vi "Match_Pressure STD.vi"(8 "abs?(F)":bool, 9 "분류코드":string, 10 "Cal STD 입력":string[][](array[string]), 11 "Condition in":string[][](array[string])) -> (0 "Cal STD(-)":string[](array[string]), 1 "Dead Weight":string[][](array[string]), 2 "Cal STD(+)":string[](array[string]), 3 "Condition out":string[][](array[string]), 4 "Cal STD(DMM)":string[][](array[string]), 5 "단위":string, 6 "Power Supply?":string, 7 "STD Name":string)   [LabVIEW 2020]
uses:
  Public/Polymorph/Data Class_2D Str.vi
  Public/Polymorph/Sort_2D Str.vi
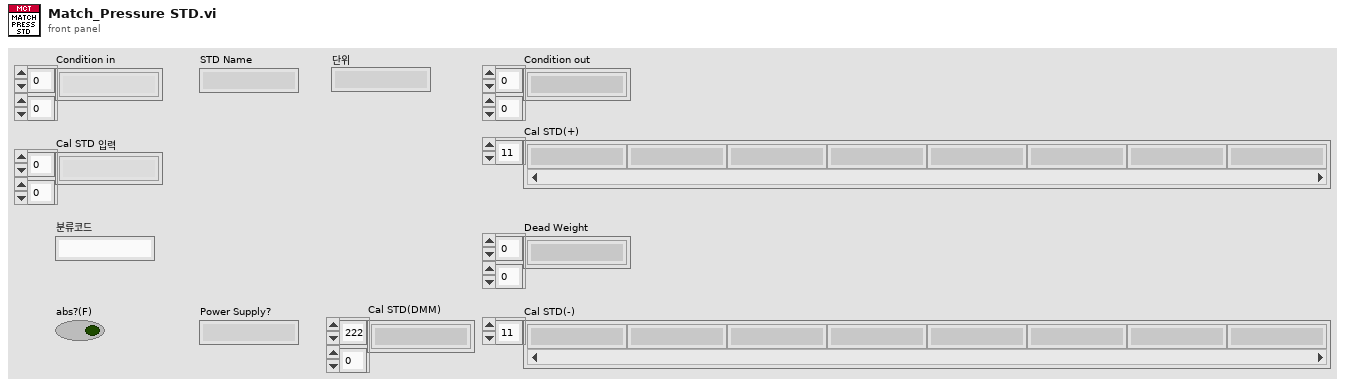
[diagram p1: front panel]
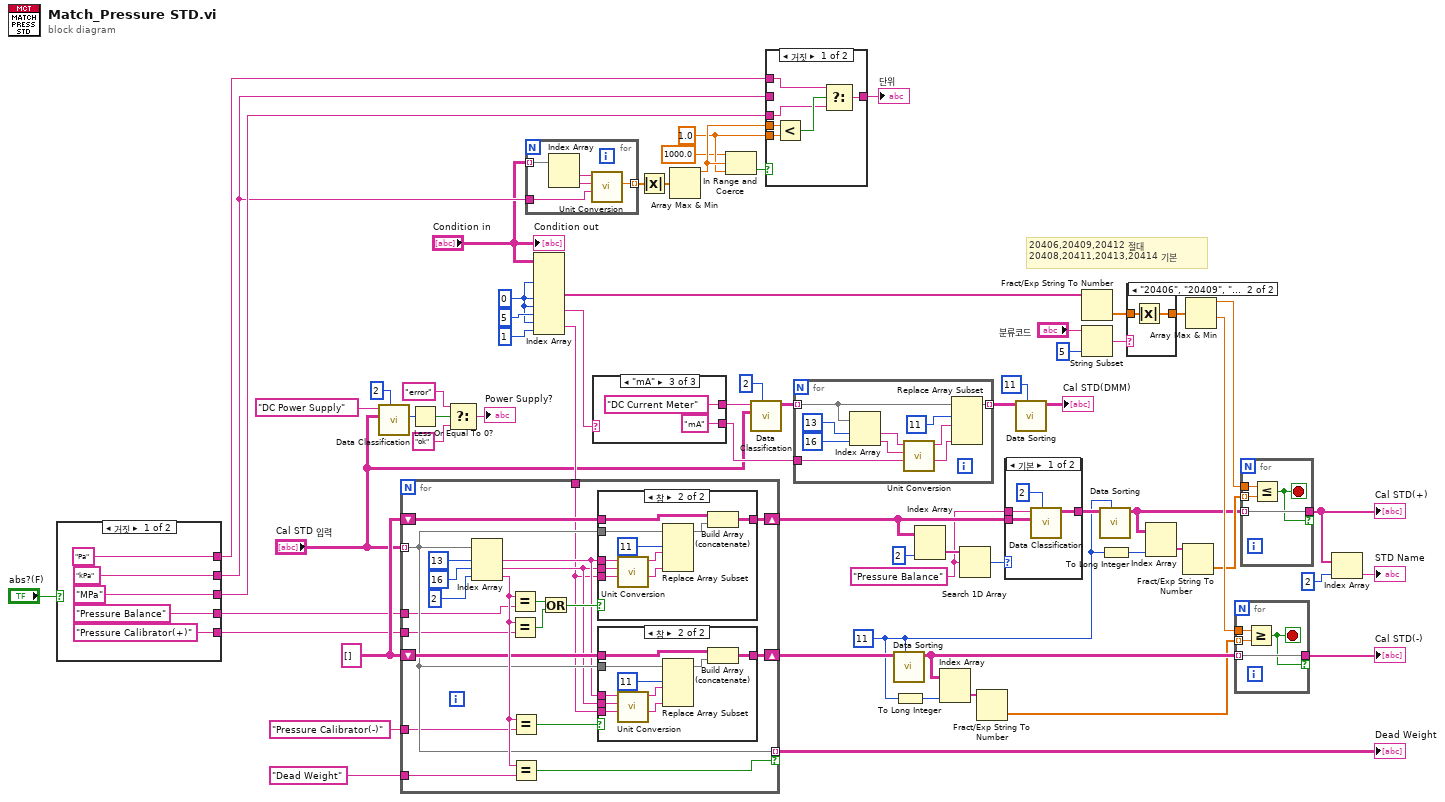
[diagram p0: block diagram]
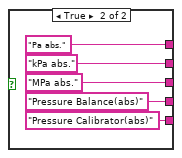
[diagram p2: hidden frame]
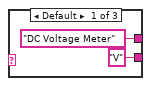
[diagram p4: hidden frame]
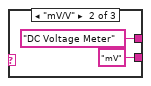
[diagram p5: hidden frame]
diagram:
  w40 = 1.0 ("하위 리미트")
  w2 = "Pressure Balance"
  w8 = u16 11 ("기준열")
  w5 = 0 ("인덱스 (행)")
  w66 = string[][] []
  # "20406,20409,20412 절대\n20408,20411,20413,20414 기본"
  n1 = case shown="거짓" "abs?(F)" {
    tunnel: ["Pressure Balance" "Pressure Balance(abs)"] -> w16
    tunnel: ["Pressure Calibrator(+)" "Pressure Calibrator(abs)"] -> w15
    tunnel: ["kPa" ("환산단위") "kPa abs." ("환산단위")] -> w12
    tunnel: ["Pa" "Pa abs."] -> w14
    tunnel: ["MPa" "MPa abs."] -> w13
    frame False {
    }
    frame True {
    }
  }
  n2 = call-poly "Data Classification.vi"("인덱스"=2, "DATA 입력"="Cal STD 입력", "검색 문자열"="DC Power Supply") -> ("행크기"=w26:i32)  [unwired: 4 in, 4 out]
  n3 = Less Or Equal To 0?(x=w26) -> (x <= 0?=w27:bool)
  n4 = Select(t="error" ("검색 문자열"), s=w27, f="ok") -> (s? t:f=→"Power Supply?":string)
  n5 = for {
    tunnel: "Condition in" -> [w81] mode=indexing
    tunnel: [w78] -> w37 mode=indexing
    tunnel: w12 -> [w77]
    n6 = Index Array(array=w81) -> (element #1=w80:string, element #2=w79:string)  [unwired: 2 in]
    n7 = call "Unit Conversion.vi"("환산단위"=w77, "입력단위"=w79, "입력값"=w80) -> ("환산값 (DBL)"=w78:dbl)  [unwired: 3 in, 5 out]
  }
  n8 = Index Array(array="Condition in", index (col) #1=w5, index (col) #2=w5, index (row) #3=w5, index (col) #3=5 ("비활성화된 인덱스 (열)"), index (row) #4=w5, index (col) #4=1 ("비활성화된 인덱스 (열)")) -> (element #2=w4:string[], element #3=w6:string, element #4=w63:string)  [unwired: 2 in, 1 out]
  n9 = for {
    tunnel: "Cal STD 입력" -> [w89] mode=indexing
    shift-right: [w98] -> w54
    shift-left: w66 -> [w97]
    tunnel: w63 -> [w86]
    tunnel: [w89] -> w65 mode=indexing if=w94
    shift-right: [w91] -> w57
    shift-left: w66 -> [w92]
    tunnel: w16 -> [w85]
    tunnel: w15 -> [w84]
    tunnel: "Pressure Calibrator(-)" -> [w83]
    tunnel: "Dead Weight" -> [w82]
    n10 = Index Array(array=w89, index #1=13 ("인덱스"), index #2=16 ("인덱스"), index #3=2 ("인덱스")) -> (element #1=w88:string, element #2=w87:string, element #3=w93:string)
    n11 = Equal?(x=w93, y=w85) -> (x = y?=w101:bool)
    n12 = Equal?(x=w93, y=w84) -> (x = y?=w100:bool)
    n13 = Equal?(x=w93, y=w83) -> (x = y?=w90:bool)
    n14 = Equal?(x=w93, y=w82) -> (x = y?=w94:bool)
    n15 = Or(x=w101, y=w100) -> (x .or. y?=w99:bool)
    n16 = case shown="참" w99 {
      tunnel: w89 -> [_ w119]
      tunnel: [w114 w124] -> w98
      tunnel: w97 -> [w114 w123]
      tunnel: w88 -> [_ w122]
      tunnel: w87 -> [_ w121]
      tunnel: w86 -> [_ w120]
      frame False {
      }
      frame True {
        n17 = call "Unit Conversion.vi"("환산단위"=w120, "입력단위"=w121, "입력값"=w122) -> ("환산단위"=w117:string, "환산값 (string)"=w118:string)  [unwired: 3 in, 4 out]
        n18 = Replace Array Subset(array=w119, new element #1=w118, index #1=11 ("인덱스"), new element #2=w117) -> (w115:string[])  [unwired: 1 in]
        n19 = Build Array (concatenate)(w123, w115) -> (w124:string[][])
      }
    }
    n20 = case shown="참" w90 {
      tunnel: w89 -> [_ w109]
      tunnel: [w103 w104] -> w91
      tunnel: w92 -> [w103 w113]
      tunnel: w88 -> [_ w112]
      tunnel: w87 -> [_ w111]
      tunnel: w86 -> [_ w110]
      frame False {
      }
      frame True {
        n21 = call "Unit Conversion.vi"("환산단위"=w110, "입력단위"=w111, "입력값"=w112) -> ("환산단위"=w107:string, "환산값 (string)"=w108:string)  [unwired: 3 in, 4 out]
        n22 = Replace Array Subset(array=w109, new element #1=w108, index #1=11 ("인덱스"), new element #2=w107) -> (w105:string[])  [unwired: 1 in]
        n23 = Build Array (concatenate)(w113, w105) -> (w104:string[][])
      }
    }
  }
  "Dead Weight" <- w65
  n24 = case shown="\"mA\"" w6 {
    tunnel: ["DC Voltage Meter" ("검색 문자열") "DC Voltage Meter" ("검색 문자열") "DC Current Meter" ("검색 문자열")] -> w34
    tunnel: ["V" "mV" "mA"] -> w32
    frame Default {
    }
    frame "mV/V" {
    }
    frame "mA" {
    }
  }
  n25 = Absolute Value(x=w37) -> (abs(x)=w42:dbl[])
  n26 = Array Max & Min(array=w42) -> (max value=w41:dbl)  [unwired: 3 out]
  n27 = In Range and Coerce(upper limit=1000.0 ("상위 리미트"), x=w41, lower limit=w40) -> (In Range?=w39:bool)  [unwired: 1 out]
  n28 = call-poly "Data Classification.vi"("인덱스"=2, "DATA 입력"="Cal STD 입력", "검색 문자열"=w34) -> ("DATA 출력"=w33:string[][])  [unwired: 4 in, 4 out]
  n29 = case shown="거짓" w39 {
    tunnel: [w133 w137] -> w36
    tunnel: w40 -> [w136 _]
    tunnel: w41 -> [w135 _]
    tunnel: w14 -> [w132 _]
    tunnel: w13 -> [w131 _]
    tunnel: w12 -> [_ w137]
    frame False {
      n30 = Less?(x=w135, y=w136) -> (x < y?=w134:bool)
      n31 = Select(t=w132, s=w134, f=w131) -> (s? t:f=w133:string)
    }
    frame True {
    }
  }
  "단위" <- w36
  n32 = for {
    tunnel: w33 -> [w143] mode=indexing
    tunnel: [w142] -> w30 mode=indexing
    tunnel: w32 -> [w147]
    n33 = Index Array(array=w143, index #1=13 ("인덱스"), index #2=16 ("인덱스")) -> (element #1=w145:string, element #2=w138:string)
    n34 = call "Unit Conversion.vi"("환산단위"=w147, "입력단위"=w138, "입력값"=w145) -> ("환산단위"=w139:string, "환산값 (string)"=w140:string)  [unwired: 3 in, 4 out]
    n35 = Replace Array Subset(array=w143, new element #1=w140, index #1=11 ("인덱스"), new element #2=w139) -> (w142:string[])  [unwired: 1 in]
  }
  n36 = call-poly "Data Sorting.vi"("기준열"=w8, "Data in"=w57) -> ("Data out"=w62:string[][])  [unwired: 8 in, 1 out]
  n37 = To Long Integer(number=w8) -> (32bit integer=w60:i32)
  n38 = Index Array(array=w54, index (col)=2 ("비활성화된 인덱스 (열)")) -> (element=w3:string[])  [unwired: 1 in]
  n39 = Index Array(array=w62, index (col)=w60) -> (element=w59:string[])  [unwired: 1 in]
  n40 = Search 1D Array(1D array=w3, element=w2) -> (index of element=w1:i32)  [unwired: 1 in]
  n41 = Fract/Exp String To Number(string=w59) -> (number=w61:dbl[])  [unwired: 3 in, 1 out]
  n42 = case shown="기본" w1 {
    tunnel: w54 -> [w151 w152]
    tunnel: [w149 w152] -> w49
    tunnel: w2 -> [w150 _]
    frame Default {
      n43 = call-poly "Data Classification.vi"("인덱스"=2, "DATA 입력"=w151, "검색 문자열"=w150) -> ("DATA 출력"=w149:string[][])  [unwired: 4 in, 4 out]
    }
    frame -1 {
    }
  }
  n44 = call-poly "Data Sorting.vi"("기준열"=u16 11, "Data in"=w30) -> ("Data out"=→"Cal STD(DMM)":string[][])  [unwired: 8 in, 1 out]
  n45 = Fract/Exp String To Number(string=w4) -> (number=w43:dbl[])  [unwired: 3 in, 1 out]
  n46 = String Subset(string="분류코드", length (rest)=5 ("길이(나머지)")) -> (substring=w19:string)  [unwired: 1 in]
  n47 = call-poly "Data Sorting.vi"("기준열"=w8, "Data in"=w49) -> ("Data out"=w50:string[][])  [unwired: 8 in, 1 out]
  n48 = To Long Integer(number=w8) -> (32bit integer=w53:i32)
  n49 = case shown="\"20406\", \"20409\", \"20412\"" w19 {
    tunnel: [w153 w154] -> w44
    tunnel: w43 -> [w153 w155]
    frame Default {
    }
    frame "20406", "20409", "20412" {
      n50 = Absolute Value(x=w155) -> (abs(x)=w154:dbl[])
    }
  }
  n51 = Index Array(array=w50, index (col)=w53) -> (element=w52:string[])  [unwired: 1 in]
  n52 = Fract/Exp String To Number(string=w52) -> (number=w51:dbl[])  [unwired: 3 in, 1 out]
  n53 = Array Max & Min(array=w44) -> (max value=w48:dbl, min value=w58:dbl)  [unwired: 2 out]
  n54 = for {
    tunnel: w58 -> [w158]
    tunnel: w62 -> [w157] mode=indexing
    tunnel: w61 -> [w159] mode=indexing
    tunnel: [w157] -> w56 if=w156
    stop <- w156 stop-if-true
    n55 = Greater Or Equal?(x=w158, y=w159) -> (x >= y?=w156:bool)
  }
  "Cal STD(-)" <- w56
  n56 = for {
    tunnel: w48 -> [w162]
    tunnel: w50 -> [w161] mode=indexing
    tunnel: w51 -> [w163] mode=indexing
    tunnel: [w161] -> w46 if=w160
    stop <- w160 stop-if-true
    n57 = Less Or Equal?(x=w162, y=w163) -> (x <= y?=w160:bool)
  }
  "Cal STD(+)" <- w46
  n58 = Index Array(array=w46, index=2 ("인덱스")) -> (element=→"STD Name":string)
  "Condition out" <- "Condition in"
